vi "TestVI_Sensors.vi"() -> ()   [LabVIEW 2018]
uses:
  <vilib>/express/express shared/transition.llb/Dynamic To Waveform Array.vi
  <vilib>/express/express signal manip/GetorSetDDTAttributes/Set DDT Attributes/SetT0.vi
  <vilib>/express/express shared/transition.llb/Waveform Array To Dynamic.vi
  <vilib>/express/express signal manip/GetorSetDDTAttributes/Set DDT Attributes/Set DDT Properties.xnode
panel:
  in  "Projects":string[](array[string])
  in  "Independent?":bool=TRUE
  in  "File Close Action":enum16{"Prompt", "Keep", "Archive", "Trash"}(ring)
  out "VI name":string="TestVI_Sensors"
  out "file path":path=path "C:/Users/aspit/Git/MHDLab/Test Data/2018-06-02/H2TC/Temp Dependence/TestVI_Sensors_200C.tdms"
  in  "File Information":T1={"Project"=0, "SubFolder"="Temp Dependence", "Filename (Meas. Description)"="200C", "Measurement number"=0} {"Project" items=["H2DT", "VaporTubes", "MaterialsTesting", "ThermalCond", "SeedFeeder"]}
  out "tdms error":errorcluster
  out "tdms file":refnum<k34>
  out "output cluster":cluster{"Sine with Uniform Noise":dynamicdata}={"Sine with Uniform Noise"=[{"t0"=timestamp(3610818365.6612945 s since 1904-01-01), "dt"=0.001, "Y"=[-0.739204421219446], "attributes"=variant("NI_ChannelName"=variant(string "Sine with Uniform Noise"), "NI_ExpIsRelativeTime"=variant(bool FALSE), "NI_ExpStartTimeStamp"=variant(timestamp timestamp(3610818355.8992944 s since 1904-01-01)), "NI_ExpTimeStamp"=variant(timestamp timestamp(3610818365.6612945 s since 1904-01-01)), "NI_ExpXDimension"=variant(string "t"))}]}
  out "Sine with Uniform Noise":dbl=-0.739204421219446
  in  "stop":bool
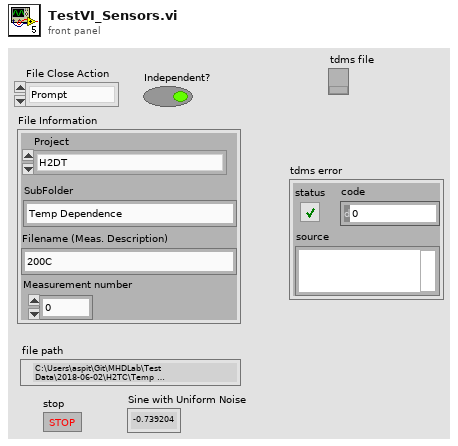
[diagram p1: front panel]
types:
  T1 = cluster{"Project":u16, "SubFolder":string, "Filename (Meas. Description)":string, "Measurement number":i32}
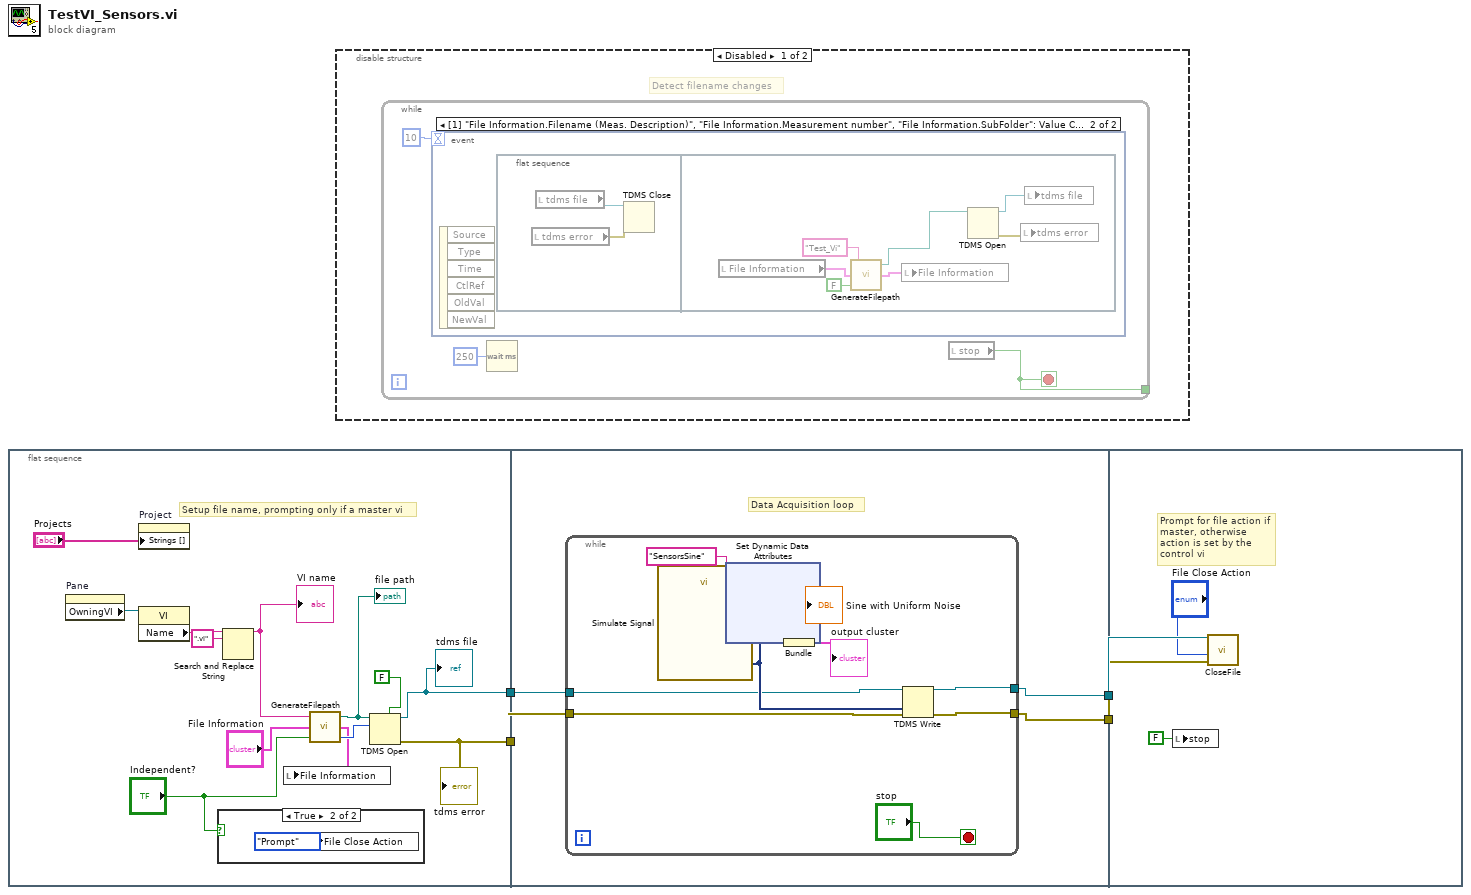
[diagram p0: block diagram]
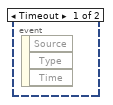
[diagram p3: hidden frame]
diagram:
  n1 = flat-sequence {
    tunnel: [w10] -> w4
    tunnel: [w9] -> w3
    tunnel: w4 -> [w22]
    tunnel: w3 -> [w21]
    tunnel: [w20] -> w2
    tunnel: [w19] -> w1
    tunnel: w2 -> [w48]
    tunnel: w1 -> [w49]
    frame #0 {
      # "Setup file name, prompting only if a master vi"
      n2 = property on="Pane" class="Pane"() -> ("OwningVI"=w16:refnum<vi>)  [unwired: 2 in, 2 out]
      n3 = property on="Project" class="Ring (strict)"("Strings []"="Projects") -> ()  [unwired: 2 in, 2 out]
      n4 = property class="VI"(reference=w16) -> ("Name"=w17:string)  [unwired: 1 in, 2 out]
      n5 = case shown="True" "Independent?" {
        frame False {
        }
        frame True {
          n6 = local write "File Close Action"(enum16{"Prompt", "Keep", "Archive", "Trash"}."Prompt" ("File Close Action")) -> ()
        }
      }
      n7 = Search and Replace String(input string=w17, search string=".vi") -> (result string=w8:string)  [unwired: 6 in, 3 out]
      "VI name" <- w8
      n8 = call "GenerateFilepath.vi"("Check for file?"="Independent?", "File Information"="File Information", "Instrument"=w8) -> ("File Action"=w14:i32, "File Information Out"=w13:T1, "File Path Out"=w7:path)
      "file path" <- w7
      n9 = local write "File Information"(w13) -> ()
      n10 = TDMS Open(5:FALSE ("create index file? (T)"), 10:w14, 11:w7) -> (0:w10:errorcluster, 3:w9:refnum<k34>)  [unwired: 4 in]
      "tdms file" <- w9
      "tdms error" <- w10
    }
    frame #1 {
      # "Data Acquisition loop"
      n11 = while {
        tunnel: [w28] -> w19
        tunnel: [w27] -> w20
        tunnel: w22 -> [w26]
        tunnel: w21 -> [w25]
        stop <- "stop" stop-if-true
        n12 = call "Simulate Signal"() -> ("Sine with Uniform Noise"=w29:dynamicdata)  [unwired: 14 in, 1 out]
        "Sine with Uniform Noise" <- w29
        n13 = xnode "Set Dynamic Data Attributes"("Signals In"=w29, "Signal Name"="SensorsSine") -> ("Signals Out"=w24:dynamicdata)  [unwired: 2 in, 1 out]
        n14 = Bundle("Signals Out"=w24) -> (→"output cluster":cluster{"Signals Out":dynamicdata})  [unwired: 1 in]
        n15 = TDMS Write(0:w25, 9:w29, 11:w26) -> (4:w28:refnum<k34>, 15:w27:errorcluster)  [unwired: 3 in, 2 out]
      }
    }
    frame #2 {
      # "Prompt for file action if master, otherwise action is set by the control vi"
      n16 = local write "stop"(FALSE ("stop")) -> ()
      n17 = call "CloseFile.vi"("error in (no error)"=w48, "Action"="File Close Action", "Refnum in"=w49) -> ()  [unwired: 8 in, 1 out]
    }
  }
  n18 = disable-structure shown="Disabled" {
    frame Disabled {
      # "Detect filename changes"
      n19 = while {
        tunnel: [w50] -> _
        stop <- w50 stop-if-true
        n20 = event shown="[1] \"File Information.Filename (Meas. Description)\", \"File Information.Measurement number\", \"File Information.SubFolder\": Value Change" {
          selector: _ -> [_ _]
          dyn-events: _ -> [_ _]
          timeout: 10 -> [_ _]
          event Timeout {
            n21 = event-data() -> ()  [unwired: 1 in, 3 out]
          }
          event "File Information.Filename (Meas. Description)", "File Information.Measurement number", "File Information.SubFolder": Value Change {
            n22 = event-data() -> ()  [unwired: 1 in, 6 out]
            n23 = flat-sequence {
              frame #0 {
                n24 = local read "tdms error"() -> (w54:errorcluster)
                n25 = local read "tdms file"() -> (w53:refnum<k34>)
                n26 = TDMS Close(8:w54, 11:w53) -> ()  [unwired: 2 out]
              }
              frame #1 {
                n27 = local read "File Information"() -> (w59:T1)
                n28 = call "GenerateFilepath.vi"("Check for file?"=FALSE, "File Information"=w59, "Instrument"="Test_Vi") -> ("File Information Out"=w61:T1, "File Path Out"=w58:path)  [unwired: 1 out]
                n29 = local write "File Information"(w61) -> ()
                n30 = TDMS Open(11:w58) -> (0:w56:errorcluster, 3:w57:refnum<k34>)  [unwired: 6 in]
                n31 = local write "tdms error"(w56) -> ()
                n32 = local write "tdms file"(w57) -> ()
              }
            }
          }
        }
        n33 = Wait (ms)(milliseconds to wait=u32 250) -> ()  [unwired: 1 out]
        n34 = local read "stop"() -> (w50:bool)
      }
    }
    frame Enabled {
    }
  }
